vi "execution class name.vi"(8 "error in":errorcluster, 11 "configuration in":refnum<class "NISE_CEF_serializable configuration.lvclass">) -> (0 "error out":errorcluster, 2 "execution class":string, 3 "configuration out":refnum<class "NISE_CEF_serializable configuration.lvclass">)   [LabVIEW 2013, in "NISE_CEF_serializable configuration.lvclass"]
uses:
  NISE_CEF_serializable configuration.lvclass
  NISE_CEF_TreeControl.lvlib
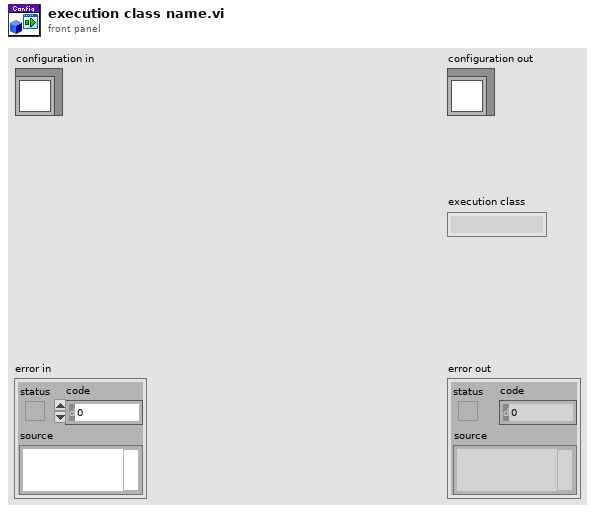
[diagram p1: front panel]
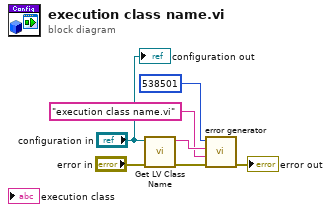
[diagram p0: block diagram]
diagram:
  n1 = call <vilib>:"Get LV Class Name.vi"("error in (no error)"="error in", "object"="configuration in") -> ("error out"=w6:errorcluster, "class name"=w5:string)  [unwired: 8 in]
  n2 = call "error generator.vi"("error in"=w6, "source"="execution class name.vi", "append error message"=w5, "error code (0)"=538501) -> ("error out"=→"error out":errorcluster)  [unwired: 5 in]
  "configuration out" <- "configuration in"
